vi "emi_Application Folder.vi"(7 "Sub Dir name":string, 11 "error in (no error)":errorcluster) -> (8 "Dir":path, 15 "error out":errorcluster)   [LabVIEW 2011]
doc: "Returns the Applications Folder. \nIf in Exe: Return the folder where Exe is located.\nIf in development: Return the folder BELOW the bottom caller(main). Below to reduce the chance of including the file in the project.\n\nAny thing in \"Sub Dir name\" is added correctly to the path.\n\nThis VI only analyses the project the first time it is called, this improves run time eficiency.\n\nIf Error in. Action performed as normal. This is nececery doe to the Run once function of this VI."
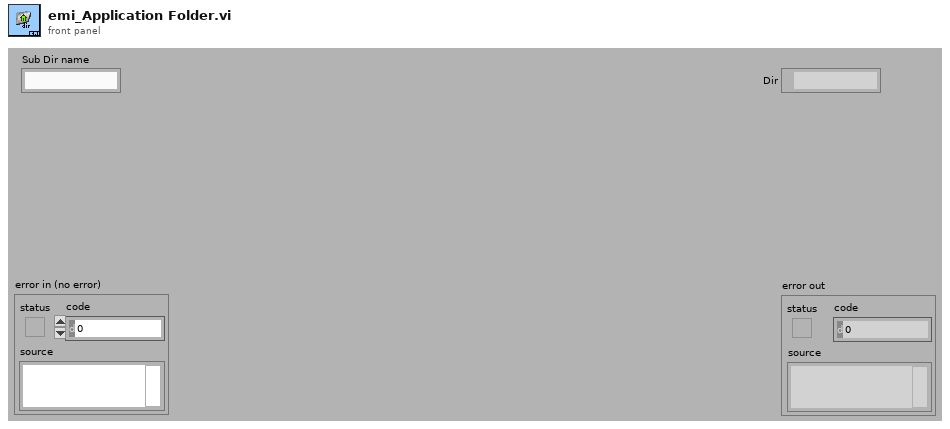
[diagram p1: front panel]
types:
  T1 = enum32{"invalid app kind", "Development System", "Run Time System", "Student Edition", "Embedded LabVIEW", "Evaluation", "Custom"}
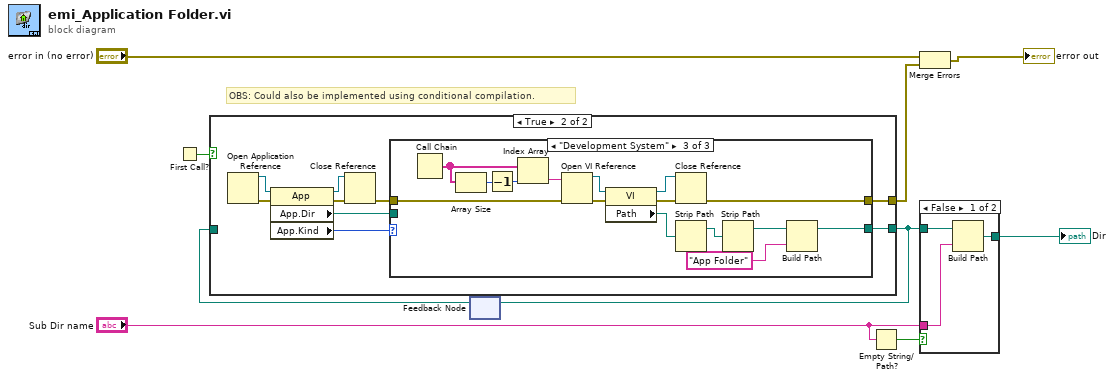
[diagram p0: block diagram]
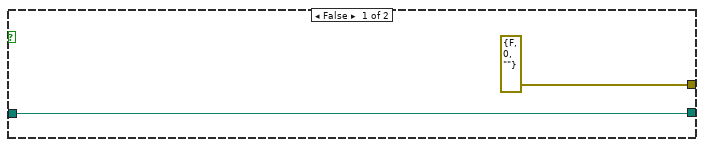
[diagram p3: hidden frame]
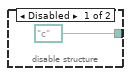
[diagram p6: hidden frame]
diagram:
  # "OBS: Could also be implemented using conditional compilation."
  n1 = First Call?() -> (First Call?: T/F=w9:bool)
  n2 = feedback #1() -> (w8:path)  [unwired: 1 in]
  n3 = case shown="True" w9 {
    tunnel: [w11 w15] -> w7
    tunnel: w8 -> [w11 _]
    tunnel: [errorcluster {"status"=FALSE, "code"=0, "source"=""} ("error out") w12] -> w1
    frame False {
    }
    frame True {
      n4 = Open Application Reference() -> (0:w20:errorcluster, 3:w19:refnum<vi>)  [unwired: 1 in, 3 out]
      n5 = property class="App"(reference=w19, error in=w20) -> (reference out=w17:refnum<vi>, error out=w18:errorcluster, "App.Dir"=w14:path, "App.Kind"=w16:T1)
      n6 = Close Reference(reference=w17, error in (no error)=w18) -> (error out=w13:errorcluster)
      n7 = case shown="\"Development System\"" w16 {
        tunnel: [w22 w24 w29] -> w15
        tunnel: w14 -> [w22 w23 _]
        tunnel: w13 -> [w21 w25 w33]
        tunnel: [w21 w25 w32] -> w12
        frame "Embedded LabVIEW" {
        }
        frame "Run Time System", Default {
          n8 = disable-structure shown="Enabled" {
            disable-tunnel: [path "c:/" ("stripped path") w27] -> w24
            disable-tunnel: w23 -> [_ w27]
            frame Disabled {
            }
            frame Enabled {
            }
          }
        }
        frame "Development System" {
          n9 = Call Chain() -> (call chain=w39:string[])
          n10 = Array Size(array=w39) -> (size(s)=w38:i32)
          n11 = Decrement(x=w38) -> (x-1=w40:i32)
          n12 = Index Array(array=w39, index=w40) -> (element=w42:string)
          n13 = Open VI Reference(vi path=w42, error in (no error)=w33) -> (vi reference=w41:refnum<vi>, error out=w37:errorcluster)  [unwired: 4 out]
          n14 = property class="VI"(reference=w41, error in=w37) -> (reference out=w34:refnum<vi>, error out=w35:errorcluster, "Path"=w36:path)
          n15 = Close Reference(reference=w34, error in (no error)=w35) -> (error out=w32:errorcluster)
          n16 = Strip Path(path=w36) -> (stripped path=w31:path)  [unwired: 1 out]
          n17 = Strip Path(path=w31) -> (stripped path=w30:path)  [unwired: 1 out]
          n18 = Build Path(base path=w30, name or relative path="App Folder") -> (appended path=w29:path)
        }
      }
    }
  }
  n19 = feedback-in #1(w7) -> ()
  n20 = Empty String/Path?(string/path="Sub Dir name") -> (empty?=w4:bool)
  n21 = Merge Errors("error in (no error)", w1) -> (→"error out":errorcluster)
  n22 = case shown="False" w4 {
    tunnel: w7 -> [w45 w46]
    tunnel: "Sub Dir name" -> [w44 _]
    tunnel: [w43 w46] -> w6
    frame False {
      n23 = Build Path(base path=w45, name or relative path=w44) -> (appended path=w43:path)
    }
    frame True {
    }
  }
  "Dir" <- w6
